vi "FPGAmain_5782_sctl_config.vi"() -> ()   [LabVIEW 2013]
uses:
  FPGA/DataMode.ctl
  FPGA/Input_5782/5782_states.ctl
  <vilib>/Platform/TimedLoop/XDataNode/timing_clust.ctl
  <vilib>/Platform/TimedLoop/XDataNode/nitl_modes.ctl
  <vilib>/Platform/TimedLoop/XDataNode/wakeup.ctl
  <vilib>/rvi/Emulation/niFpgaSctlEmulationGetInTimedLoop.vi
  <vilib>/rvi/Emulation/niFpgaEmulationReportErrorSimple.vi
  <vilib>/rvi/Emulation/niFpgaGetClockAttributes.vi
  <vilib>/rvi/Emulation/niFpgaCriticalErrorInLSC.vi
  <vilib>/rvi/eio/common/nirviEmuTemplateMethod_errors.vi
  <vilib>/rvi/DataTransferAndStorage/Register/Emulation/niFpgaRegisterEmulationFpgaImpl.vi
  <instcachedir>/0/niFpgaRegisterEmulationFpgaImpl_DCF4BC0110594B98B44A971D60CEEC4D.lvgen/niFpgaRegisterEmulationFpgaImpl_DCF4BC0110594B98B44A971D60CEEC4D_003.vi
  <vilib>/rvi/DataTransferAndStorage/Container/Common/niFpgaContainerGetUniqueNameForEmu.vi
  <instcachedir>/0/niFpgaRegisterEmulationFpgaImpl_DCF4BC0110594B98B44A971D60CEEC4D.lvgen/niFpgaRegisterEmulationFpgaImpl_DCF4BC0110594B98B44A971D60CEEC4D_016.vi
  <instcachedir>/0/niFpgaRegisterEmulationFpgaImpl_DCF4BC0110594B98B44A971D60CEEC4D.lvgen/niFpgaRegisterEmulationFpgaImpl_DCF4BC0110594B98B44A971D60CEEC4D_010.vi
  <instcachedir>/0/niFpgaRegisterEmulationFpgaImpl_DCF4BC0110594B98B44A971D60CEEC4D.lvgen/niFpgaRegisterEmulationFpgaImpl_DCF4BC0110594B98B44A971D60CEEC4D_011.vi
  <instcachedir>/0/niFpgaRegisterEmulationFpgaImpl_DCF4BC0110594B98B44A971D60CEEC4D.lvgen/niFpgaRegisterEmulationFpgaImpl_DCF4BC0110594B98B44A971D60CEEC4D_012.vi
  <instcachedir>/0/niFpgaRegisterEmulationFpgaImpl_DCF4BC0110594B98B44A971D60CEEC4D.lvgen/niFpgaRegisterEmulationFpgaImpl_DCF4BC0110594B98B44A971D60CEEC4D_009.vi
  <vilib>/rvi/FIFO/Fifo_Resource/nirvififoEmulationReadFpgaImpl.vi
  <vilib>/rvi/interface/RandomDataEmulation/nirviRandomDataMultiElementFPGAFIFO.vi
  <instcachedir>/0/nirviRandomDataMultiElementFPGAFIFO_F2B80EDE0D7944A08478D8D26097D4DB.lvgen/nirviRandomDataMultiElementFPGAFIFO_F2B80EDE0D7944A08478D8D26097D4DB_005.vi
  <vilib>/rvi/interface/RandomDataEmulation/niFpgaRandomDataHandleErrors.vi
  <instcachedir>/0/niFpgaRegisterEmulationFpgaImpl_DCF4BC0110594B98B44A971D60CEEC4D.lvgen/niFpgaRegisterEmulationFpgaImpl_DCF4BC0110594B98B44A971D60CEEC4D_013.vi
  <vilib>/rvi/interface/RandomDataEmulation/nirviRandomDataFPGAFIFO.vi
  <vilib>/rvi/FIFO/Fifo_Resource/nirvififoEmulationWriteFpgaImpl.vi
  <vilib>/Platform/TimedLoop/XDataNode/XDataNode.xnode
  <vilib>/eio/EIONode/EIONode.xnode
  <vilib>/rvi/DataTransferAndStorage/Container/XNode/niFpgaContainer.xnode
  <vilib>/rvi/DataTransferAndStorage/Register/Emulation/niFpgaRegisterEmulation.vi
  <vilib>/rvi/FIFO/Fifo_Resource/nirvififoEmulationRead.vi
  <vilib>/rvi/interface/RandomDataEmulation/nirviRandomDataFpgaMultiElementTemplate.vi
  <vilib>/rvi/interface/RandomDataEmulation/nirviRandomDataFpgaReadWriteTemplate.vi
  <vilib>/rvi/FIFO/Fifo_Resource/nirvififoEmulationWrite.vi
  <vilib>/Platform/TimedLoop/XDataNode/XDNodeRunTimeDep.lvlib
panel:
  in  "AM phase":fxp<+,64,64>
  in  "delay phase":fxp<+,64,64>
  in  "User Command Commit":bool
  in  "User Command":u8
  out "User Command Idle":bool
  out "User Command Status":u8
  in  "User Data 0":u8
  in  "User Data 1":u8
  out "PLL Locked":bool
  out "User Error":bool
  out "Configured?":bool
  in  "Continuous":bool
  in  "5782 record length":u16=4000 caption="Samples Per Trigger" min=1 step=1
  in  "Trigger Acquisition":bool
  out "IO Module\\Trigger Input":bool
  in  "Downsample":fxp<+,8,8>=1.0
  in  "new coeffs":bool
  in  "FIR coeffs":fxp<+/-,18,18>[](array[numeric])
  in  "CIC Gain":fxp<+/-,32,1>=0.00390625 format="%#_32g"
  in  "Acquisition running":bool
  in  "Phase output":fxp<+,64,64>[](array[numeric])=[0.0, 0.0, 0.0, 0.0, 0.0, 0.0, 0.0, 0.0]
  in  "Simulated phase 5782":fxp<+,64,64>[](array[numeric])=[0.0, 0.0]
  in  "Mode":T1
  in  "Phase 5782":fxp<+,64,64>[](array[numeric])=[0.0, 0.0]
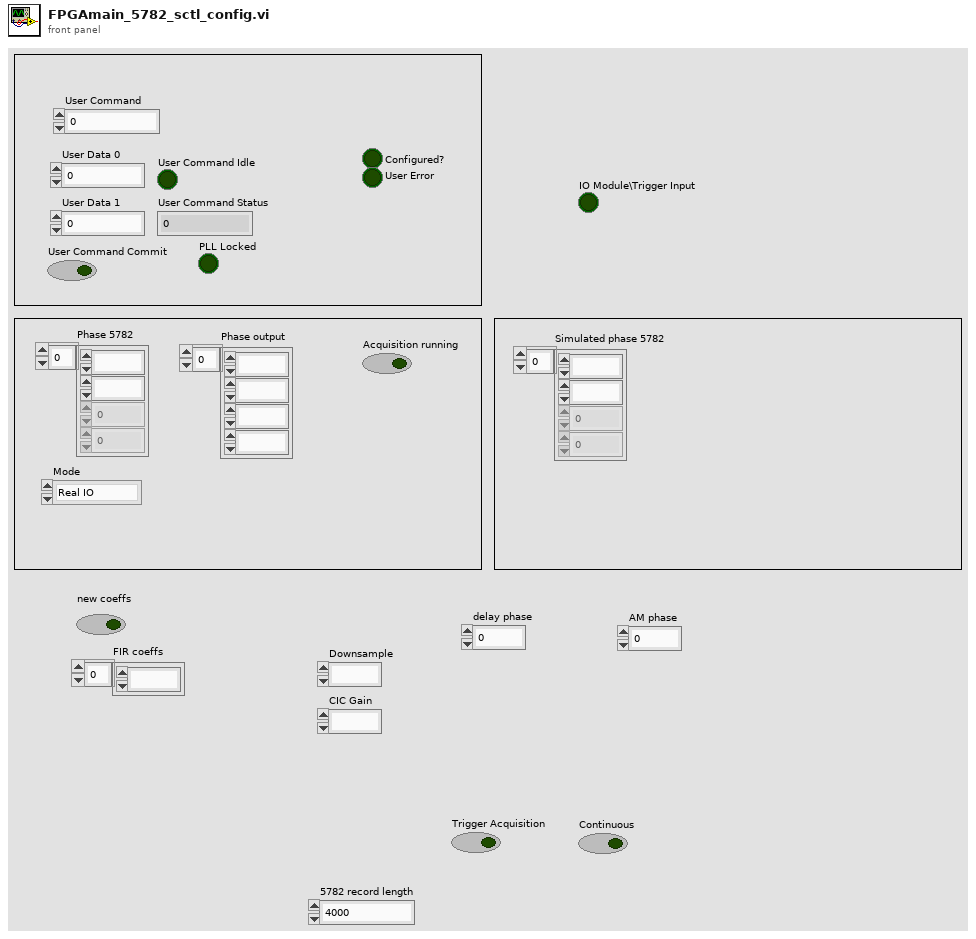
[diagram p1: front panel]
types:
  T1 = typedef "DataMode.ctl" = enum16{"Real IO", "Simulated"}
  T2 = typedef "5782_states.ctl" = enum8{"Wait for trigger", "Acquisition", "Send record length", "Quiet period"}
  T3 = typedef "XDNodeRunTimeDep.lvlib/timing_clust.ctl" = cluster{"Expected End [f-1]":u64, "Actual End [f-1]":u64, "Finished Late? [f-1]":bool, "Expected End [i-1]":u64, "Actual End [i-1]":u64, "Finished Late? [i-1]":bool, "Expected Start [i]":u64, "Actual Start [i]":u64, "Expected Start [f]":u64, "Actual Start [f]":u64, "Source Name":string, "Structure Name":string, "Period":i64, "Deadline":i64, "Offset":i64, "Start":i64, "Priority":i32, "Timeout":i32, "Mode":T4, "Wakeup Reason":T5, "Error":errorcluster, "Source Type":string, "Secondary Source Type":string, "Global End Time":u64, "Global Start Time":u64, "Frame Duration":u64, "Iteration Duration":u64, "Assigned CPU":i32, "I/O Scan Engine Mode":u32}
  T4 = typedef "XDNodeRunTimeDep.lvlib/nitl_modes.ctl" = enum32{"No Change", "Process missed periods, maintain original phase", "Discard missed periods, maintain original phase", "Process missed periods, ignore original phase", "Discard missed periods, ignore original phase"}
  T5 = typedef "XDNodeRunTimeDep.lvlib/wakeup.ctl" = enum32{"Normal", "Aborted", "Asynchronous wakeup", "Timing source error", "Timed loop error", "Timeout"}
  T6 = typedef "I16 array size 2.ctl" = i16[]
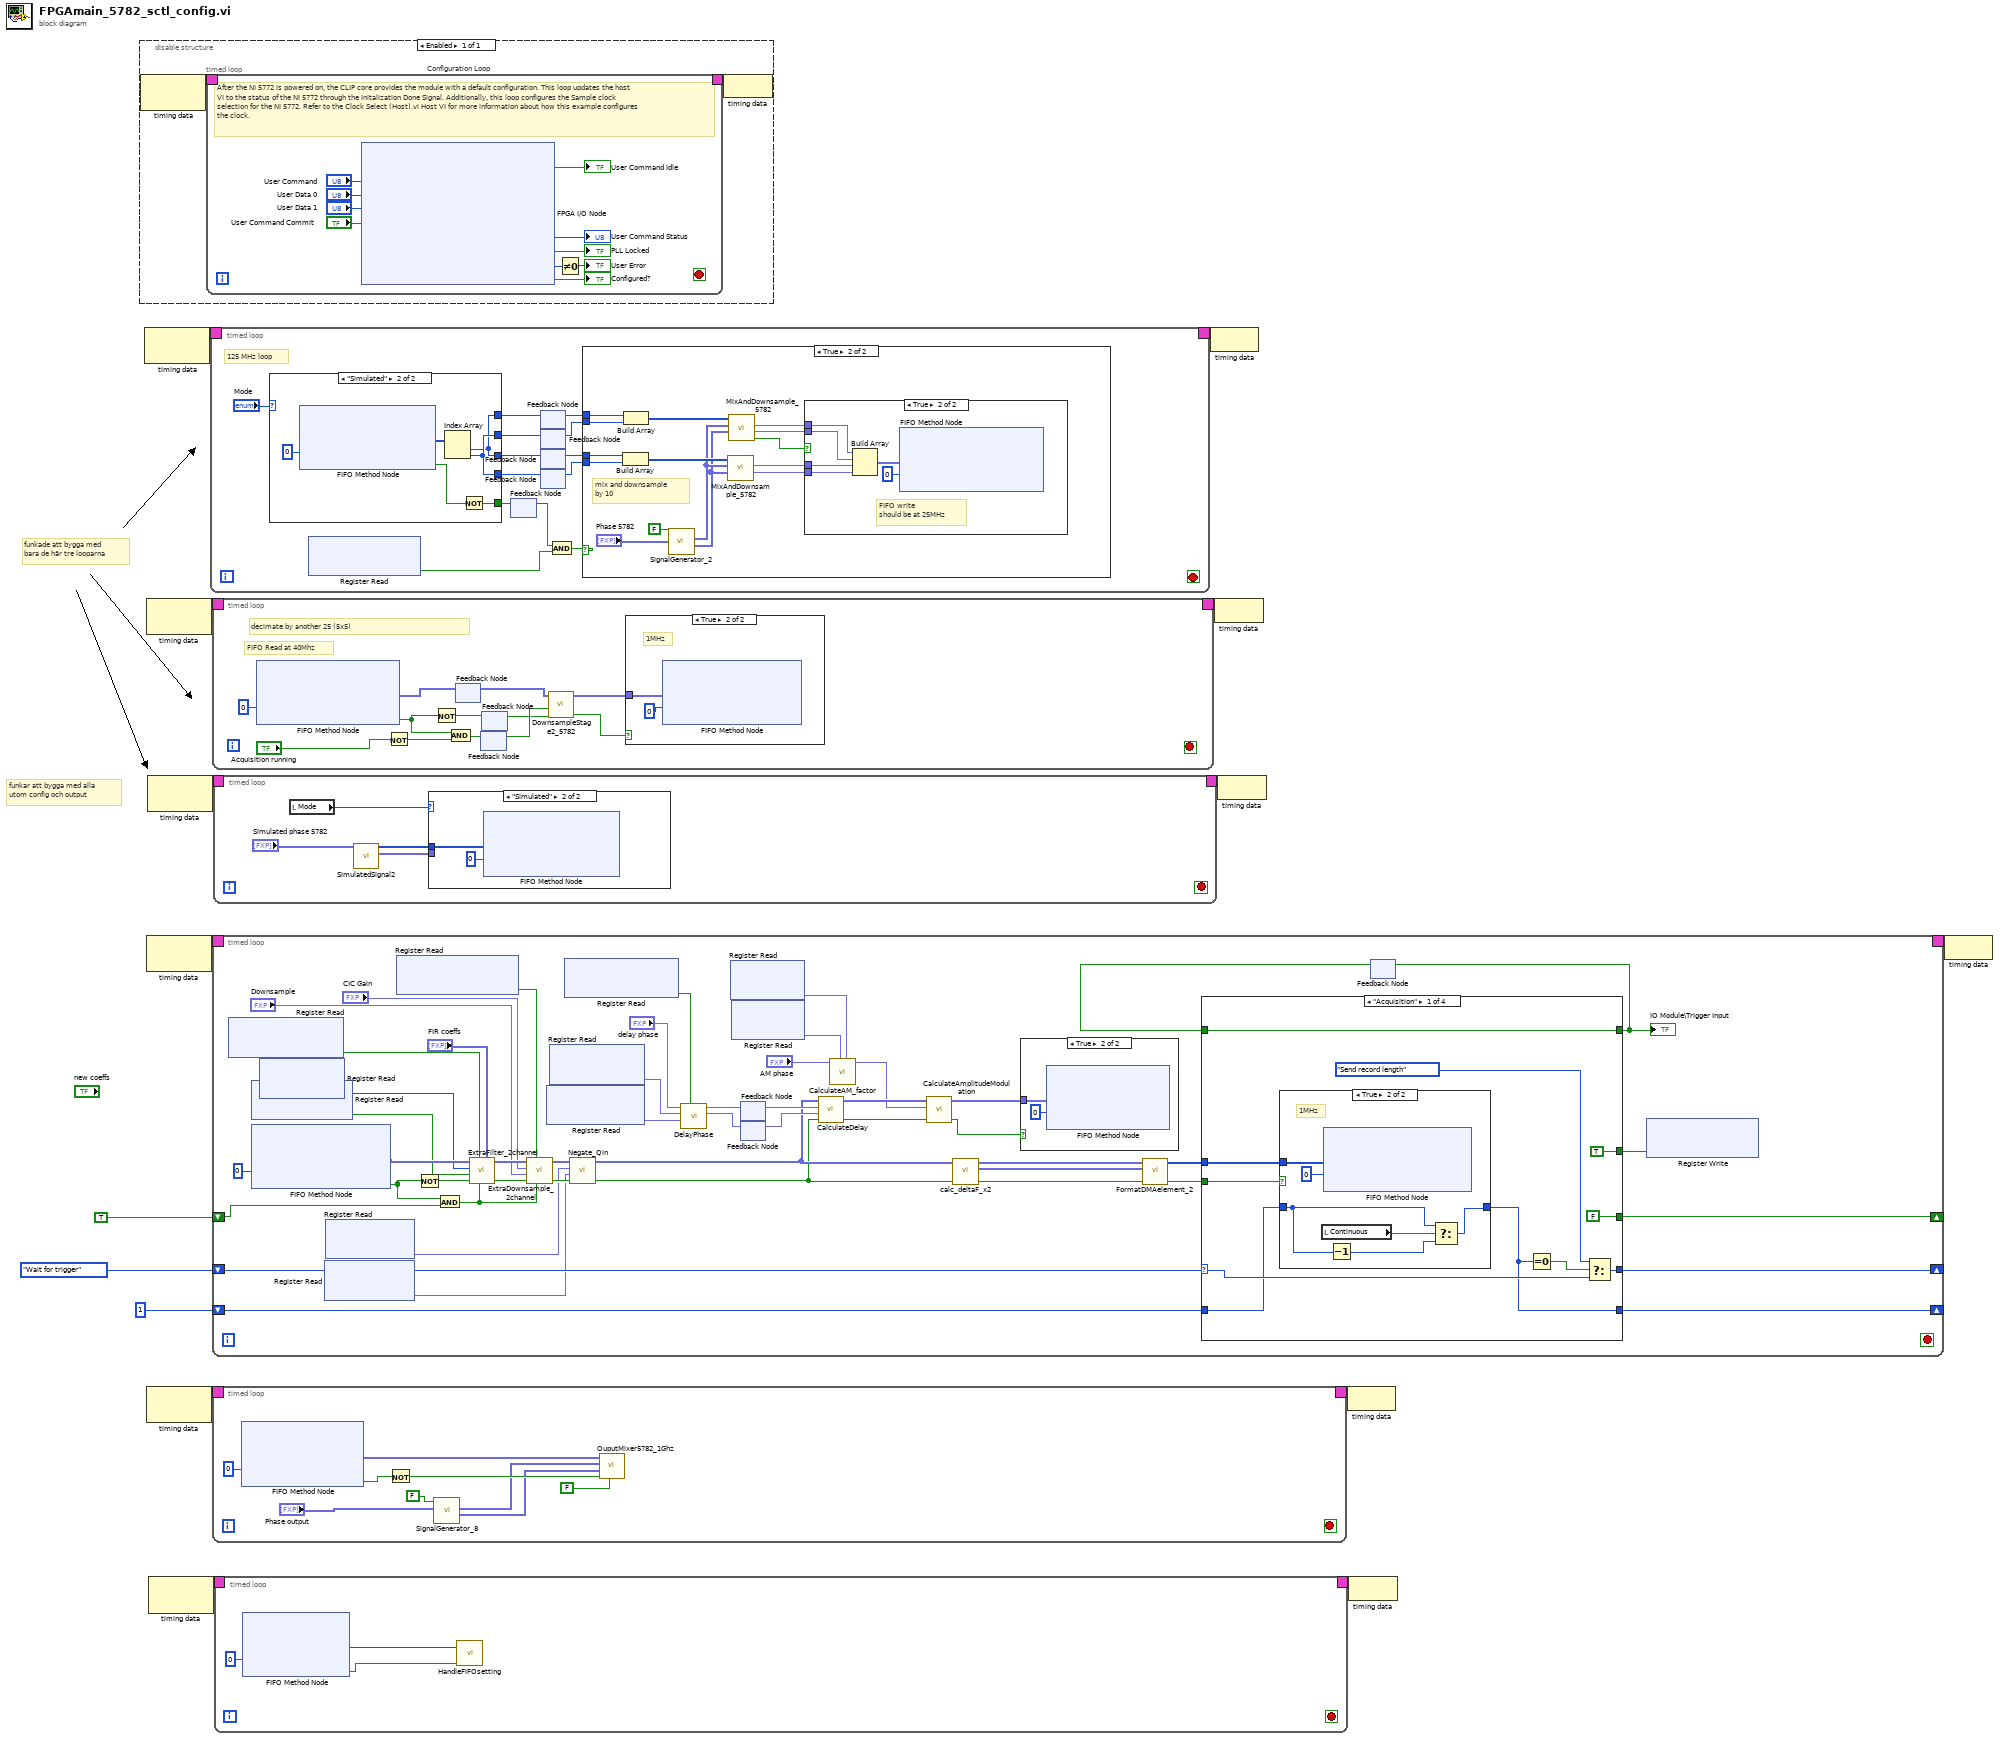
[diagram p0: block diagram]
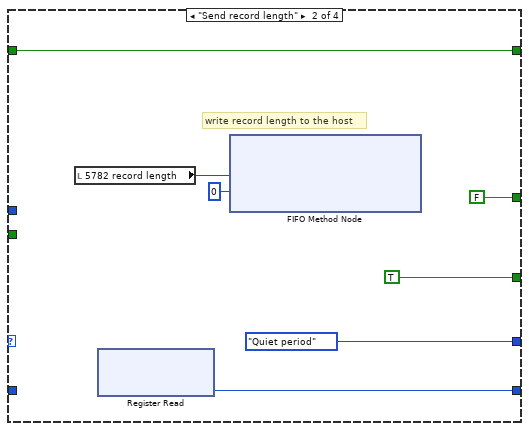
[diagram p4: hidden frame]
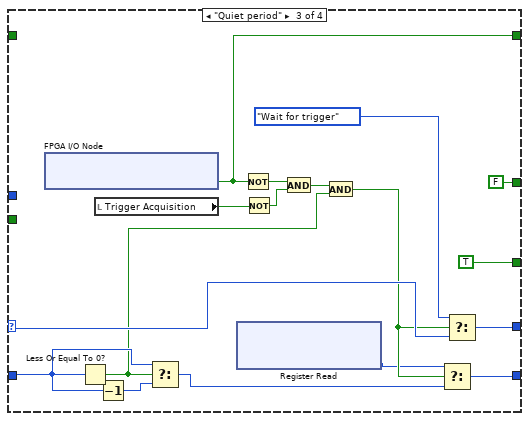
[diagram p5: hidden frame]
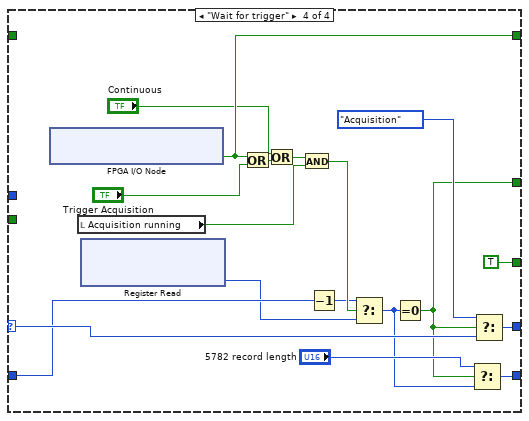
[diagram p6: hidden frame]
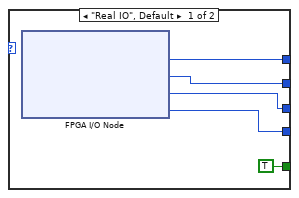
[diagram p9: hidden frame]
diagram:
  # "funkar att bygga med alla\nutom config och output"
  # "funkade att bygga med\nbara de här tre looparna"
  n1 = disable-structure shown="Enabled" {
    frame Enabled {
      n2 = node-c288() -> (w17:T3)  [unwired: 1 in]
      n3 = timed-loop "Configuration Loop" {
        timing: w17 -> [_]
        timing-out: [_] -> w16
        stop <- _ stop-if-true
        # "After the NI 5772 is powered on, the CLIP core provides the module with a default configuration. This loop updates the host VI to the status of the NI 5772 through the Initalization Done Signal. Additionally, this loop configures the Sample clock selection for the NI 5772. Refer to the Clock Select (Host).vi Host VI for more information about how this example configures the clock."
        n4 = xnode "FPGA I/O Node"("IO Module\\User Command"="User Command", "IO Module\\User Data 0"="User Data 0", "IO Module\\User Data 1"="User Data 1", "IO Module\\User Command Commit"="User Command Commit") -> ("IO Module\\User Command Idle"=→"User Command Idle":bool, "IO Module\\User Command Status"=→"User Command Status":u8, "IO Module\\PLL Locked"=→"PLL Locked":bool, "IO Module\\User Error"=w23:u8, "IO Module\\Initialization Done"=→"Configured?":bool)  [unwired: 9 in, 9 out]
        n5 = Not Equal To 0?(x=w23) -> (x != 0?=→"User Error":bool)
      }
      n6 = node-c288(w16) -> ()
    }
  }
  n7 = node-c288() -> (w11:T3)  [unwired: 1 in]
  n8 = node-c288() -> (w15:T3)  [unwired: 1 in]
  n9 = node-c288() -> (w9:T3)  [unwired: 1 in]
  n10 = node-c288() -> (w2:T3)  [unwired: 1 in]
  n11 = node-c288() -> (w13:T3)  [unwired: 1 in]
  n12 = node-c288() -> (w4:T3)  [unwired: 1 in]
  n13 = timed-loop {
    timing: w11 -> [_]
    timing-out: [_] -> w10
    stop <- _ stop-if-true
    # "125 MHz loop"
    n14 = case shown="\"Simulated\"" "Mode" {
      tunnel: [w70 w73] -> w42
      tunnel: [w69 w74] -> w40
      tunnel: [w68 w73] -> w38
      tunnel: [w67 w74] -> w35
      tunnel: [TRUE w71] -> w34
      frame "Real IO", Default {
        n15 = xnode "FPGA I/O Node"() -> ("IO Module\\AI 0 N-1"=w70:i16, "IO Module\\AI 0 N"=w69:i16, "IO Module\\AI 1 N-1"=w68:i16, "IO Module\\AI 1 N"=w67:i16)  [unwired: 4 in, 4 out]
      }
      frame "Simulated" {
        n16 = xnode ("FIFO Method Node")("Timeout"=0) -> ("Element"=w75:i16[], "Timed Out?"=w72:bool)  [unwired: 1 in, 1 out]
        n17 = Index Array(array=w75) -> (element #1=w73:i16, element #2=w74:i16)  [unwired: 2 in]
        n18 = Not(x=w72) -> (.not. x?=w71:bool)
      }
    }
    n19 = xnode ("Register Read")() -> ("Data"=w32:bool)  [unwired: 1 in, 1 out]
    n20 = feedback #1() -> (w33:bool)  [unwired: 1 in]
    n21 = feedback-in #1(w34) -> ()
    n22 = feedback #2() -> (w41:i16)  [unwired: 1 in]
    n23 = feedback-in #2(w42) -> ()
    n24 = feedback #3() -> (w39:i16)  [unwired: 1 in]
    n25 = feedback-in #3(w40) -> ()
    n26 = feedback #4() -> (w37:i16)  [unwired: 1 in]
    n27 = feedback-in #4(w38) -> ()
    n28 = feedback #5() -> (w36:i16)  [unwired: 1 in]
    n29 = feedback-in #5(w35) -> ()
    n30 = And(x=w33, y=w32) -> (x .and. y?=w43:bool)
    n31 = case shown="True" w43 {
      tunnel: w41 -> [_ w50]
      tunnel: w39 -> [_ w49]
      tunnel: w37 -> [_ w48]
      tunnel: w36 -> [_ w47]
      frame False {
      }
      frame True {
        # "mix and downsample\nby 10"
        n32 = Build Array(w48, w47) -> (w59:i16[])
        n33 = Build Array(w50, w49) -> (w46:i16[])
        n34 = call "SignalGenerator_2.vi"("Phase"="Phase 5782", "reset"=FALSE) -> ("Sine out"=w51:fxp<+/-,16,0>[], "Cosine out"=w52:fxp<+/-,16,0>[])  [unwired: 8 in]
        n35 = call "MixAndDownsample_5782.vi"("Sine in"=w51, "Cosine in"=w52, "Signal Input"=w59) -> ("Q out"=w54:fxp<+/-,16,14>, "I out"=w55:fxp<+/-,16,14>)  [unwired: 6 in, 1 out]
        n36 = call "MixAndDownsample_5782.vi"("Sine in"=w51, "Cosine in"=w52, "Signal Input"=w46) -> ("data valid"=w56:bool, "Q out"=w57:fxp<+/-,16,14>, "I out"=w58:fxp<+/-,16,14>)  [unwired: 6 in]
        n37 = case shown="True" w56 {
          tunnel: w57 -> [_ w65]
          tunnel: w58 -> [_ w62]
          tunnel: w55 -> [_ w61]
          tunnel: w54 -> [_ w60]
          frame False {
          }
          frame True {
            # "FIFO write\nshould be at 25MHz"
            n38 = Build Array(w62, w65, w61, w60) -> (w64:fxp<+/-,16,14>[])
            n39 = xnode ("FIFO Method Node")("Element"=w64, "Timeout"=0) -> ()  [unwired: 1 in, 2 out]
          }
        }
      }
    }
  }
  n40 = timed-loop {
    timing: w15 -> [_]
    timing-out: [_] -> w14
    stop <- _ stop-if-true
    # "FIFO Read at 40Mhz"
    # "decimate by another 25 (5x5)"
    n41 = xnode ("FIFO Method Node")("Timeout"=0) -> ("Element"=w84:fxp<+/-,16,14>[], "Timed Out?"=w86:bool)  [unwired: 1 in, 1 out]
    n42 = Not(x="Acquisition running") -> (.not. x?=w87:bool)
    n43 = Not(x=w86) -> (.not. x?=w80:bool)
    n44 = And(x=w86, y=w87) -> (x .and. y?=w82:bool)
    n45 = feedback #6() -> (w83:fxp<+/-,16,14>[])  [unwired: 1 in]
    n46 = feedback-in #6(w84) -> ()
    n47 = feedback #7() -> (w81:bool)  [unwired: 1 in]
    n48 = feedback-in #7(w82) -> ()
    n49 = feedback #8() -> (w79:bool)  [unwired: 1 in]
    n50 = feedback-in #8(w80) -> ()
    n51 = call "DownsampleStage2_5782.vi"("valid in"=w79, "reset"=w81, "Data in"=w83) -> ("valid out"=w88:bool, "data out"=w89:fxp<+/-,16,14>[])  [unwired: 7 in]
    n52 = case shown="True" w88 {
      tunnel: w89 -> [_ w91]
      frame False {
      }
      frame True {
        # "1MHz"
        n53 = xnode ("FIFO Method Node")("Element"=w91, "Timeout"=0) -> ()  [unwired: 1 in, 2 out]
      }
    }
  }
  n54 = timed-loop {
    timing: w9 -> [_]
    timing-out: [_] -> w8
    shift-right: [w142] -> _
    shift-left: 5782_states."Wait for trigger" ("5782 states") -> [w144]
    shift-right: [w141] -> _
    shift-left: u16 1 ("trigger samples") -> [w143]
    shift-right: [w127] -> _
    shift-left: TRUE -> [w130]
    stop <- _ stop-if-true
    n55 = xnode ("Register Read")() -> ("Data"=w105:bool)  [unwired: 1 in, 1 out]
    n56 = xnode ("Register Read")() -> ("Data"=w95:bool)  [unwired: 1 in, 1 out]
    n57 = xnode ("FIFO Method Node")("Timeout"=0) -> ("Element"=w132:fxp<+/-,16,14>[], "Timed Out?"=w131:bool)  [unwired: 1 in, 1 out]
    n58 = xnode ("Register Read")() -> ("Data"=w96:i32)  [unwired: 1 in, 1 out]
    n59 = xnode ("Register Read")() -> ("Data"=w103:fxp<+/-,16,14>)  [unwired: 1 in, 1 out]
    n60 = xnode ("Register Read")() -> ("Data"=w104:fxp<+/-,16,14>)  [unwired: 1 in, 1 out]
    n61 = xnode ("Register Read")() -> ("Data"=w97:bool)  [unwired: 1 in, 1 out]
    n62 = Not(x=w131) -> (.not. x?=w137:bool)
    n63 = And(x=w131, y=w130) -> (x .and. y?=w139:bool)
    n64 = call "ExtraFilter_2channel.vi"(5:"new coeffs"="FIR coeffs", "reset"=w139, 7:"new coeffs"=w105, "valid in"=w137, "enable filter"=w95, "new shift"=w96, "Data in"=w132) -> ("valid out"=w138:bool, "Data out"=w136:fxp<+/-,16,14>[])  [unwired: 3 in]
    n65 = call "ExtraDownsample_2channel.vi"("reset"=w139, "Set downsample"=w97, "valid in"=w138, "Downsample"="Downsample", "CIC Gain"="CIC Gain", "Data in"=w136) -> ("valid out"=w122:bool, "Data out"=w123:fxp<+/-,16,14>[])  [unwired: 4 in]
    n66 = xnode ("Register Read")() -> ("Data"=w98:fxp<+/-,16,0>)  [unwired: 1 in, 1 out]
    n67 = xnode ("Register Read")() -> ("Data"=w99:fxp<+/-,16,0>)  [unwired: 1 in, 1 out]
    n68 = xnode ("Register Read")() -> ("Data"=w100:bool)  [unwired: 1 in, 1 out]
    n69 = call "Negate_Qin.vi"("valid in"=w122, "DC offset chan 1"=w103, "DC offset chan 0"=w104, "Data in"=w123) -> ("valid out"=w108:bool, "Data out"=w114:fxp<+/-,16,14>[])  [unwired: 6 in]
    n70 = call "DelayPhase.vi"("Use fixed delay"=w100, "fixed cos_fi"=w98, "fixed sin fi"=w99, "delay phase"="delay phase") -> ("cos_fi"=w111:fxp<+/-,16,0>, "sin fi"=w112:fxp<+/-,16,0>)  [unwired: 6 in]
    n71 = xnode ("Register Read")() -> ("Data"=w102:fxp<+/-,16,2>)  [unwired: 1 in, 1 out]
    n72 = xnode ("Register Read")() -> ("Data"=w101:fxp<+/-,16,2>)  [unwired: 1 in, 1 out]
    n73 = feedback-in #9(w112) -> ()
    n74 = feedback #9() -> (w121:fxp<+/-,16,0>)  [unwired: 1 in]
    n75 = feedback #10() -> (w120:fxp<+/-,16,0>)  [unwired: 1 in]
    n76 = feedback-in #10(w111) -> ()
    n77 = call "CalculateDelay.vi"("input valid"=w108, "cos_fi"=w120, "sin fi"=w121, "Data in"=w114) -> ("output valid"=w118:bool, "Data out"=w119:fxp<+/-,16,14>[])  [unwired: 6 in]
    n78 = call "CalculateAM_factor.vi"("b_am"=w102, "a_am"=w101, "AM phase"="AM phase") -> ("AM_factor"=w115:fxp<+/-,16,2>)  [unwired: 7 in, 1 out]
    n79 = call "CalculateAmplitudeModulation.vi"("input valid"=w118, "AM_factor"=w115, "Data in"=w119) -> ("output valid"=w116:bool, "Data out"=w117:fxp<+/-,16,14>[])  [unwired: 7 in]
    n80 = call "calc_deltaF_x2.vi"("valid in"=w108, "Data in"=w114) -> ("valid out"=w107:bool, "deltaF"=w106:fxp<+/-,32,30>[], "Data out"=w109:fxp<+/-,16,14>[])  [unwired: 7 in]
    n81 = case shown="True" w116 {
      tunnel: w117 -> [_ w145]
      frame False {
      }
      frame True {
        n82 = xnode ("FIFO Method Node")("Element"=w145, "Timeout"=0) -> ()  [unwired: 1 in, 2 out]
      }
    }
    n83 = call "FormatDMAelement_2.vi"("valid in"=w107, "deltaF"=w106, "Data in"=w109) -> ("valid out"=w128:bool, "Element"=w129:u64[])  [unwired: 7 in]
    n84 = feedback #11() -> (w125:bool)  [unwired: 1 in]
    n85 = case shown="\"Acquisition\"" w144 {
      selector: w144 -> [w157 _ w187 w206]
      tunnel: w143 -> [w153 _ w175 w193]
      tunnel: [w156 5782_states."Quiet period" ("5782 states") w186 w205] -> w142
      tunnel: [w150 w165 w188 w204] -> w141
      tunnel: w129 -> [w151 _ _ _]
      tunnel: w128 -> [w152 _ _ _]
      tunnel: [FALSE TRUE TRUE TRUE] -> w127
      tunnel: [TRUE FALSE ("5782 triggered") FALSE ("5782 triggered") w197] -> w126
      tunnel: [w149 w166 w177 w196] -> w124
      tunnel: w125 -> [w149 w166 _ _]
      frame "Acquisition" {
        n86 = case shown="True" w152 {
          tunnel: w151 -> [_ w164]
          tunnel: [w158 w161] -> w150
          tunnel: w153 -> [w158 w159]
          frame False {
          }
          frame True {
            # "1MHz"
            n87 = local read "Continuous"() -> (w162:bool)
            n88 = xnode ("FIFO Method Node")("Element"=w164, "Timeout"=0) -> ()  [unwired: 1 in, 2 out]
            n89 = Decrement(x=w159) -> (x-1=w160:u16)
            n90 = Select(t=w159, s=w162, f=w160) -> (s? t:f=w161:u16)
          }
        }
        n91 = Equal To 0?(x=w150) -> (x = 0?=w154:bool)
        n92 = Select(t=5782_states."Send record length" ("5782 states"), s=w154, f=w157) -> (s? t:f=w156:T2)
      }
      frame "Send record length" {
        # "write record length to the host"
        n93 = local read "5782 record length"() -> (w168:u16)
        n94 = xnode ("Register Read")() -> ("Data"=w165:u16)  [unwired: 1 in, 1 out]
        n95 = xnode ("FIFO Method Node")("Element"=w168, "Timeout"=0) -> ()  [unwired: 1 in, 2 out]
      }
      frame "Quiet period" {
        n96 = xnode "FPGA I/O Node"() -> ("IO Module\\Trigger Input"=w177:bool)  [unwired: 1 in, 1 out]
        n97 = Less Or Equal To 0?(x=w175) -> (x <= 0?=w174:bool)
        n98 = local read "Trigger Acquisition"() -> (w183:bool)
        n99 = Decrement(x=w175) -> (x-1=w176:u16)
        n100 = Select(t=w175, s=w174, f=w176) -> (s? t:f=w173:u16)
        n101 = xnode ("Register Read")() -> ("Data"=w172:u16)  [unwired: 1 in, 1 out]
        n102 = Not(x=w177) -> (.not. x?=w182:bool)
        n103 = Not(x=w183) -> (.not. x?=w181:bool)
        n104 = And(x=w182, y=w181) -> (x .and. y?=w180:bool)
        n105 = And(x=w180, y=w174) -> (x .and. y?=w185:bool)
        n106 = Select(t=w172, s=w185, f=w173) -> (s? t:f=w188:u16)
        n107 = Select(t=5782_states."Wait for trigger" ("5782 states"), s=w185, f=w187) -> (s? t:f=w186:T2)
      }
      frame "Wait for trigger" {
        n108 = xnode "FPGA I/O Node"() -> ("IO Module\\Trigger Input"=w196:bool)  [unwired: 1 in, 1 out]
        n109 = local read "Acquisition running"() -> (w198:bool)
        n110 = xnode ("Register Read")() -> ("Data"=w189:u16)  [unwired: 1 in, 1 out]
        n111 = Or(x=w196, y="Trigger Acquisition") -> (x .or. y?=w192:bool)
        n112 = Or(x="Continuous", y=w192) -> (x .or. y?=w190:bool)
        n113 = And(x=w190, y=w198) -> (x .and. y?=w199:bool)
        n114 = Decrement(x=w193) -> (x-1=w194:u16)
        n115 = Select(t=w194, s=w199, f=w189) -> (s? t:f=w195:u16)
        n116 = Equal To 0?(x=w195) -> (x = 0?=w197:bool)
        n117 = Select(t="5782 record length", s=w197, f=w195) -> (s? t:f=w204:u16)
        n118 = Select(t=5782_states."Acquisition" ("5782 states"), s=w197, f=w206) -> (s? t:f=w205:T2)
      }
    }
    "IO Module\\Trigger Input" <- w124
    n119 = feedback-in #11(w124) -> ()
    n120 = xnode ("Register Write")("Data"=w126) -> ()  [unwired: 1 in, 1 out]
  }
  n121 = timed-loop {
    timing: w2 -> [_]
    timing-out: [_] -> w1
    stop <- _ stop-if-true
    n122 = xnode ("FIFO Method Node")("Timeout"=0) -> ("Element"=w213:fxp<+/-,16,14>[], "Timed Out?"=w216:bool)  [unwired: 1 in, 1 out]
    n123 = Not(x=w216) -> (.not. x?=w212:bool)
    n124 = call "SignalGenerator_8.vi"("Phase"="Phase output", "reset"=FALSE) -> ("Sine out"=w209:fxp<+/-,16,0>[], "Cosine out"=w210:fxp<+/-,16,0>[])  [unwired: 8 in]
    n125 = call "OuputMixer5782_1Ghz.vi"("reset"=FALSE, "valid in"=w212, "Sine in"=w209, "Cosine in"=w210, "Data in"=w213) -> ()  [unwired: 5 in, 2 out]
  }
  n126 = timed-loop {
    timing: w13 -> [_]
    timing-out: [_] -> w12
    stop <- _ stop-if-true
    n127 = local read "Mode"() -> (w223:T1)
    n128 = call "SimulatedSignal2.vi"("Phase"="Simulated phase 5782") -> ("dummy do not use"=w220:fxp<+/-,16,0>[], "output"=w222:T6)  [unwired: 9 in]
    n129 = case shown="\"Simulated\"" w223 {
      tunnel: w222 -> [_ w224]
      tunnel: w220 -> [_ _]
      frame "Real IO", Default {
      }
      frame "Simulated" {
        n130 = xnode ("FIFO Method Node")("Element"=w224, "Timeout"=0) -> ()  [unwired: 1 in, 2 out]
      }
    }
  }
  n131 = timed-loop {
    timing: w4 -> [_]
    timing-out: [_] -> w3
    stop <- _ stop-if-true
    n132 = xnode ("FIFO Method Node")("Timeout"=0) -> ("Element"=w229:u64, "Timed Out?"=w228:bool)  [unwired: 1 in, 1 out]
    n133 = call "HandleFIFOsetting.vi"("timed out"=w228, "Value"=w229) -> ()  [unwired: 10 in]
  }
  n134 = node-c288(w10) -> ()
  n135 = node-c288(w14) -> ()
  n136 = node-c288(w12) -> ()
  n137 = node-c288(w1) -> ()
  n138 = node-c288(w3) -> ()
  n139 = node-c288(w8) -> ()
